vi "connect.vi"(8 "error in (no error)":errorcluster, 11 "TCPClient in":refnum<class "TCPClient.lvclass">) -> (0 "error out":errorcluster, 3 "TCPClient out":refnum<class "TCPClient.lvclass">)   [LabVIEW 2016, in "TCPClient.lvclass"]
uses:
  TCPClient.lvclass
  TCPClient.lvclass/TCPClient.ctl
  common_ascii_tcp/TCPClient/TCPClient.lvclass
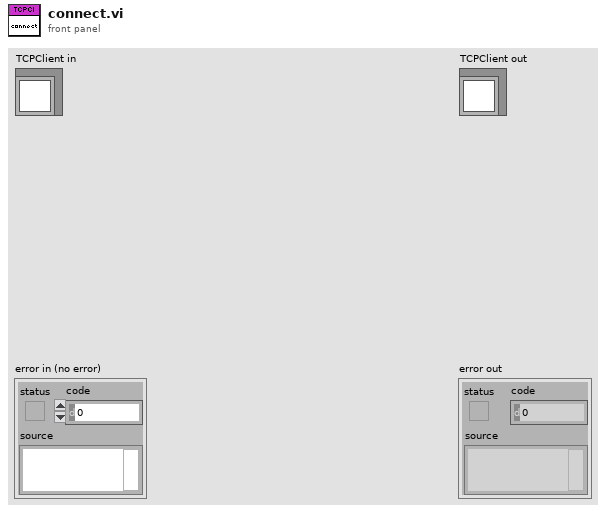
[diagram p1: front panel]
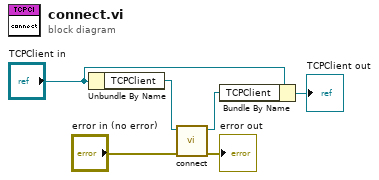
[diagram p0: block diagram]
diagram:
  n1 = Unbundle By Name("TCPClient in") -> ("TCPClient"=w1:refnum<class "TCPClient.lvclass">)
  n2 = call-dynamic "connect.vi"("error in (no error)"="error in (no error)", "TCPClient in"=w1) -> ("error out"=→"error out":errorcluster, "TCPClient out"=w3:refnum<class "TCPClient.lvclass">)  [unwired: 8 in]
  n3 = Bundle By Name(cluster="TCPClient in", "TCPClient"=w3) -> (→"TCPClient out":refnum<class "TCPClient.lvclass">)
